vi "Terminal-LoadSpectrum-ExecuteRow.vi"(11 "索引 (行)":u32) -> (0 "error IO":errorcluster, 3 "结果":T1(ring))   [LabVIEW 2014]
uses:
  Terminal-Global-SetValues.vi
panel:
  in  "停止":bool caption="启动"
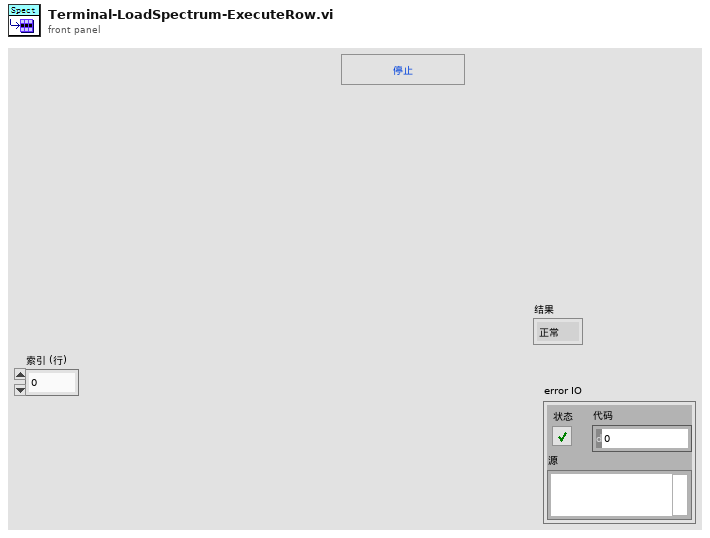
[diagram p1: front panel]
types:
  T1 = enum16{"正常", "内部异常", "修改载荷谱", "外部异常", "外部停止", "其他"}
  T2 = cluster{"报警级别":string, "报警系统":string, "报警详情":string, "备注":string}
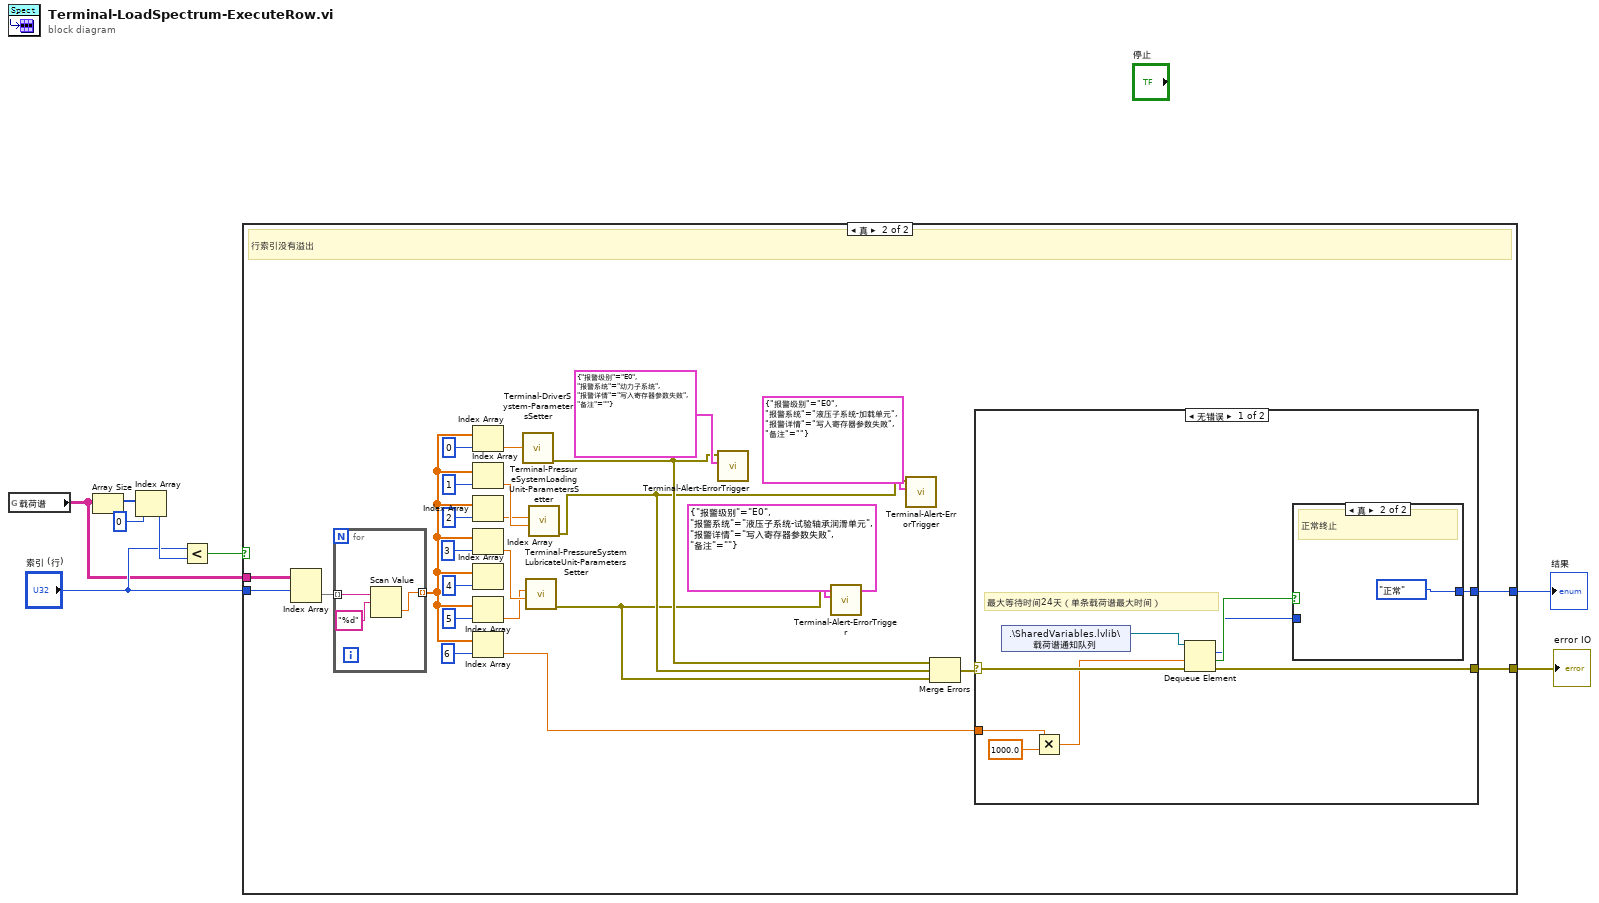
[diagram p0: block diagram]
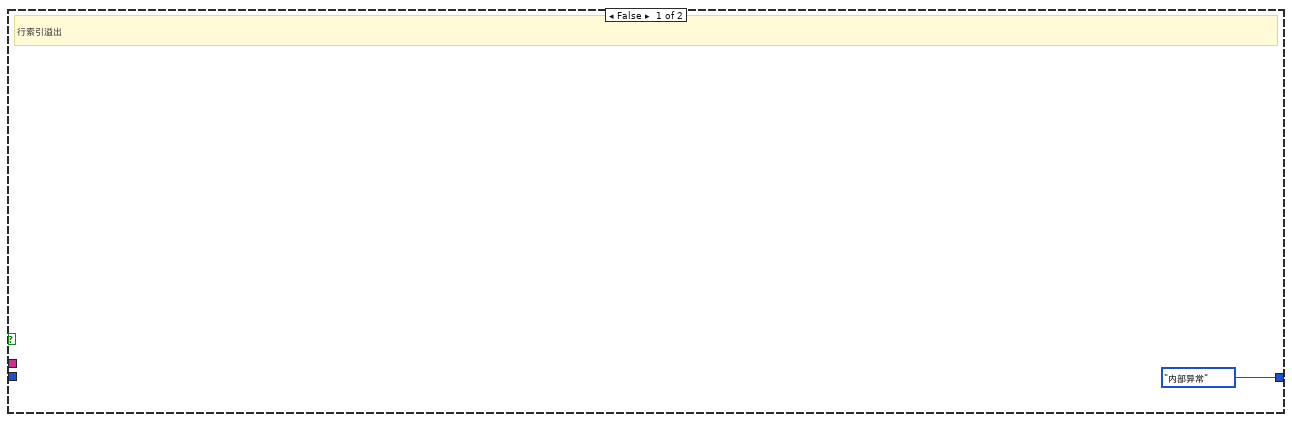
[diagram p2: hidden frame]
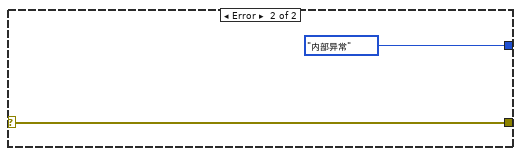
[diagram p4: hidden frame]
diagram:
  n1 = global read "Terminal-Global-SetValues.vi" "载荷谱"() -> (w2:string[][])
  n2 = Array Size(array=w2) -> (size(s)=w6:i32[])
  n3 = Index Array(array=w6, index=0 ("索引")) -> (element=w4:i32)
  n4 = Less?(x="索引 (行)", y=w4) -> (x < y?=w1:bool)
  n5 = case shown="真" w1 {
    tunnel: [_ w14] -> w8
    tunnel: [T1."内部异常" w12] -> w7
    tunnel: "索引 (行)" -> [_ w11]
    tunnel: w2 -> [_ w10]
    frame False {
      # "行索引溢出"
    }
    frame True {
      # "行索引没有溢出"
      n6 = Index Array(array=w10, index (row)=w11) -> (element=w35:string[])  [unwired: 1 in]
      n7 = for {
        tunnel: w35 -> [w51] mode=indexing
        tunnel: [w49] -> w34 mode=indexing
        n8 = Scan Value(string=w51, format string="%d" ("格式字符串")) -> (value=w49:dbl)  [unwired: 1 in, 1 out]
      }
      n9 = Index Array(array=w34, index=0 ("索引")) -> (element=w26:dbl)
      n10 = Index Array(array=w34, index=1 ("索引")) -> (element=w25:dbl)
      n11 = Index Array(array=w34, index=2 ("索引")) -> (element=w24:dbl)
      n12 = Index Array(array=w34, index=3 ("索引")) -> (element=w23:dbl)
      n13 = Index Array(array=w34, index=4 ("索引")) -> ()  [unwired: 1 out]
      n14 = Index Array(array=w34, index=5 ("索引")) -> (element=w22:dbl)
      n15 = Index Array(array=w34, index=6 ("索引")) -> (element=w13:dbl)
      n16 = call "Terminal-DriverSystem-ParametersSetter.vi"("转速"=w26) -> ("error out"=w18:errorcluster)  [unwired: 10 in]
      n17 = call "Terminal-PressureSystemLubricateUnit-ParametersSetter.vi"("供油润滑温度T"=w23, "供油流量L"=w22) -> ("error out"=w16:errorcluster)  [unwired: 9 in]
      n18 = call "Terminal-PressureSystemLoadingUnit-ParametersSetter.vi"("轴向载荷F2"=w25, "径向载荷F1"=w24) -> ("error out"=w17:errorcluster)  [unwired: 9 in]
      n19 = call "Terminal-Alert-ErrorTrigger.vi"("报警信息"=T2 {"报警级别"="E0", "报警系统"="动力子系统", "报警详情"="写入寄存器参数失败", "备注"=""}, "error in (no error)"=w18) -> ()  [unwired: 10 in]
      n20 = call "Terminal-Alert-ErrorTrigger.vi"("报警信息"=T2 {"报警级别"="E0", "报警系统"="液压子系统-试验轴承润滑单元", "报警详情"="写入寄存器参数失败", "备注"=""}, "error in (no error)"=w16) -> ()  [unwired: 10 in]
      n21 = call "Terminal-Alert-ErrorTrigger.vi"("报警信息"=T2 {"报警级别"="E0", "报警系统"="液压子系统-加载单元", "报警详情"="写入寄存器参数失败", "备注"=""}, "error in (no error)"=w17) -> ()  [unwired: 10 in]
      n22 = Merge Errors(w18, w17, w16) -> (w15:errorcluster)
      n23 = case shown="无错误" w15 {
        selector: w15 -> [w44 w48]
        tunnel: [w43 w48] -> w14
        tunnel: w13 -> [w36 _]
        tunnel: [w40 T1."内部异常"] -> w12
        frame No Error {
          # "最大等待时间24天（单条载荷谱最大时间）"
          n24 = shared-variable ".\\SharedVariables.lvlib\\载荷谱通知队列"() -> (w39:refnum<queue>)  [unwired: 1 in, 1 out]
          n25 = Multiply(x=w36, y=1000.0) -> (x*y=w37:dbl)
          n26 = Dequeue Element(queue=w39, timeout in ms (-1)=w37, error in (no error)=w44) -> (element=w41:T1, timed out?=w42:bool, error out=w43:errorcluster)  [unwired: 1 out]
          n27 = case shown="真" w42 {
            tunnel: w41 -> [w45 _]
            tunnel: [w45 T1."正常"] -> w40
            frame False {
              # "人为或异常终止"
            }
            frame True {
              # "正常终止"
            }
          }
        }
        frame Error {
        }
      }
    }
  }
  "error IO" <- w8
  "结果" <- w7
